vi "magnet initialize.vi"(8 "error in (no error)":errorcluster) -> (0 "error out":errorcluster)   [LabVIEW 2016]
uses:
  E:/C/Users/Desktop/VTI LabView IS20160920/config.vi
panel:
  out "Numeric 2":dbl format="%#_13g"
  out "Numeric":dbl format="%#_13g"
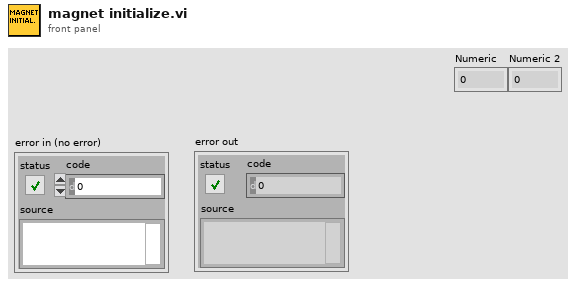
[diagram p1: front panel]
types:
  T1 = cluster{"GPIB address":i16, "GPIB bus":i16, "connection ID":refnum<k5>, "IP":string, "Active Comm Interface":u16, "Serial Port":refnum<visa-resource-name>, "Programmer Type":u16}
  T2 = cluster{"error":bool, "code":i32, "source":string}
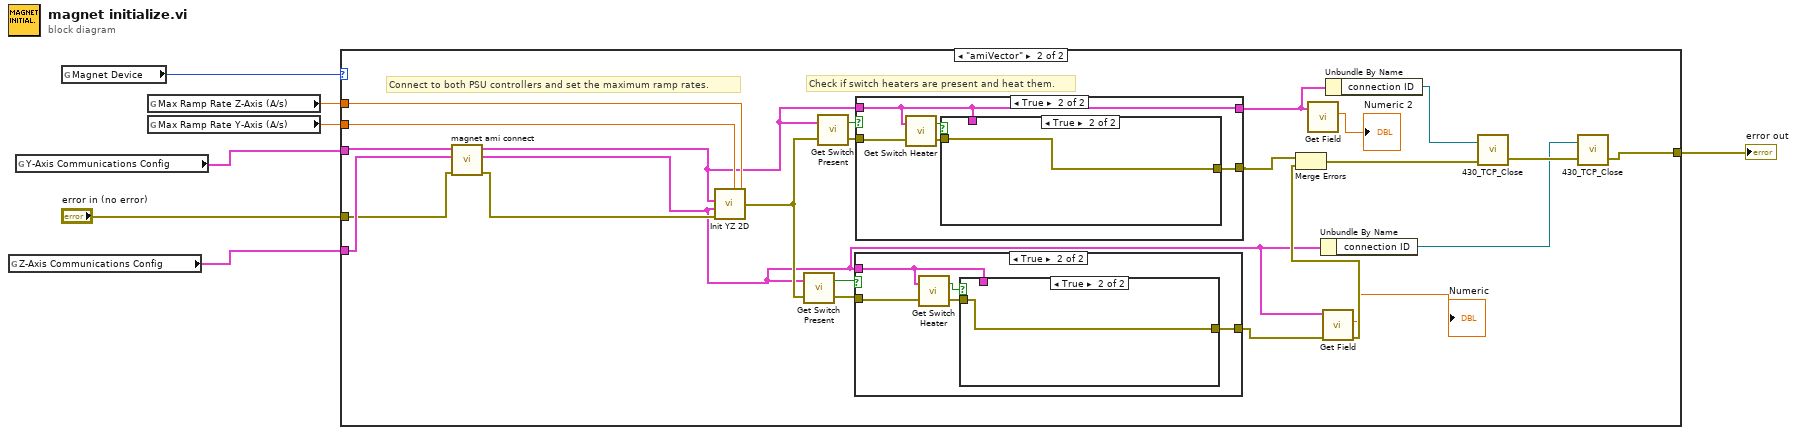
[diagram p0: block diagram]
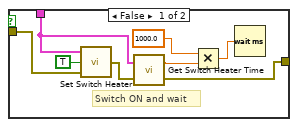
[diagram p4: hidden frame]
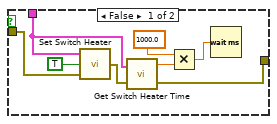
[diagram p6: hidden frame]
diagram:
  n1 = global read "config.vi" "Z-Axis Communications Config"() -> (w5:T1)
  n2 = global read "config.vi" "Y-Axis Communications Config"() -> (w4:T1)
  n3 = global read "config.vi" "Magnet Device"() -> (w7:enum16{"ips120", "amiVector"})
  n4 = global read "config.vi" "Max Ramp Rate Z-Axis (A/s)"() -> (w2:dbl)
  n5 = global read "config.vi" "Max Ramp Rate Y-Axis (A/s)"() -> (w3:dbl)
  n6 = case shown="\"amiVector\"" w7 {
    tunnel: "error in (no error)" -> [w8 w19]
    tunnel: w5 -> [_ w20]
    tunnel: w4 -> [_ w21]
    tunnel: w3 -> [_ w31]
    tunnel: w2 -> [_ w32]
    tunnel: [w8 w25] -> w1
    frame "ips120", Default {
    }
    frame "amiVector" {
      # "Check if switch heaters are present and heat them."
      # "Connect to both PSU controllers and set the maximum ramp rates."
      n7 = call "magnet ami connect.vi"("error in (no error)"=w19, "Z-Axis Communications Config"=w20, "Y-Axis Communications Config"=w21) -> ("error out"=w18:errorcluster, "Z-Axis Communications Config Out"=w12:T1, "Y-Axis Communications Config Out"=w17:T1)  [unwired: 6 in]
      n8 = call "Init YZ 2D.vi"("Max Ramp Rate Z-axis"=w32, "Max Ramp Rate Y-axis"=w31, "error in"=w18, "Z-Axis Communications Config"=w12, "Y-Axis Communications Config"=w17) -> ("error out"=w26:T2)  [unwired: 5 in]
      n9 = call "Get Switch Present.vi"("error in"=w26, "Communications Config"=w12) -> ("error out"=w30:T2, "Switch Present?"=w29:bool)
      n10 = call "Get Switch Present.vi"("error in"=w26, "Communications Config"=w17) -> ("error out"=w28:T2, "Switch Present?"=w27:bool)
      n11 = case shown="True" w29 {
        tunnel: w30 -> [w49 w52]
        tunnel: w12 -> [_ w51]
        tunnel: [w49 w50] -> w14
        frame False {
        }
        frame True {
          n12 = call "Get Switch Heater.vi"("error in"=w52, "Communications Config"=w51) -> ("error out"=w54:T2, "Switch Heater Indicator"=w53:bool)
          n13 = case shown="True" w53 {
            tunnel: w54 -> [w61 w63]
            tunnel: w51 -> [w57 _]
            tunnel: [w55 w63] -> w50
            frame False {
              n14 = call "Set Switch Heater.vi"("error in"=w61, "Switch Heater Control"=TRUE, "Communications Config"=w57) -> ("error out"=w56:T2)
              n15 = call "Get Switch Heater Time.vi"("error in"=w56, "Communications Config"=w57) -> ("error out"=w55:T2, "Switch Heating Time (secs)"=w58:dbl)
              n16 = Multiply(x=1000.0 ("y"), y=w58) -> (x*y=w60:dbl)
              n17 = Wait (ms)(milliseconds to wait=w60) -> ()  [unwired: 1 out]
            }
            frame True {
            }
          }
        }
      }
      n18 = case shown="True" w27 {
        tunnel: w28 -> [w33 w38]
        tunnel: w17 -> [w34 w39]
        tunnel: [w34 w39] -> w10
        tunnel: [w33 w35] -> w15
        frame False {
        }
        frame True {
          n19 = call "Get Switch Heater.vi"("error in"=w38, "Communications Config"=w39) -> ("error out"=w37:T2, "Switch Heater Indicator"=w36:bool)
          n20 = case shown="True" w36 {
            tunnel: w37 -> [w46 w48]
            tunnel: [w42 w48] -> w35
            tunnel: w39 -> [w40 _]
            frame False {
              # "Switch ON and wait"
              n21 = call "Set Switch Heater.vi"("error in"=w46, "Switch Heater Control"=TRUE, "Communications Config"=w40) -> ("error out"=w41:T2)
              n22 = call "Get Switch Heater Time.vi"("error in"=w41, "Communications Config"=w40) -> ("error out"=w42:T2, "Switch Heating Time (secs)"=w43:dbl)
              n23 = Multiply(x=1000.0 ("y"), y=w43) -> (x*y=w45:dbl)
              n24 = Wait (ms)(milliseconds to wait=w45) -> ()  [unwired: 1 out]
            }
            frame True {
            }
          }
        }
      }
      n25 = call "Get Field.vi"("Z-Axis Communications Config"=w10) -> ("Field(T)"=→"Numeric 2":dbl)  [unwired: 5 in, 2 out]
      n26 = Unbundle By Name(w12) -> ("connection ID"=w22:refnum<k5>)
      n27 = call "Get Field.vi"("Z-Axis Communications Config"=w12, "error in"=w14) -> ("Field(T)"=→"Numeric":dbl, "error out"=w13:T2)  [unwired: 4 in, 1 out]
      n28 = Merge Errors(w15, w13) -> (w16:errorcluster)
      n29 = Unbundle By Name(w10) -> ("connection ID"=w23:refnum<k5>)
      n30 = call "430_TCP_Close.vi"("error in (no error)"=w16, "connection ID"=w23) -> ("error out"=w24:errorcluster)  [unwired: 1 out]
      n31 = call "430_TCP_Close.vi"("error in (no error)"=w24, "connection ID"=w22) -> ("error out"=w25:errorcluster)  [unwired: 1 out]
    }
  }
  "error out" <- w1
